vi "Example - Basic IPS-Use_In_Loops.vi"(0 "Connection Details":T5={"VISA resource name"="", "Comms Layer"=enum."Ethernet TCP/IP", "IP Address"="", "Serial Configuration"={"Baud Rate"=9600, "Parity"=0, "Data Bits"=8, "Stop Bits"=10, "Flow Control"=0}, "ISOBUS address"=-1} {"Serial Configuration"."Flow Control" items=["None", "XON/XOFF", "RTS/CTS", "XON/XOFF & RTS/CTS", "DTR/DSR", "XON/XOFF & DTR/DSR"]; "Serial Configuration"."Stop Bits" items=["1.0"=10, "2.0"=20]; "Serial Configuration"."Data Bits" items=["7"=7, "8"=8]; "Serial Configuration"."Parity" items=["None", "Odd", "Even"]; "Serial Configuration"."Baud Rate" items=["300"=300, "600"=600, "1200"=1200, "2400"=2400, "4800"=4800, "9600"=9600, "19200"=19200]}, 1 "Axis Group":string(combo)="GRPZ", 2 "ID Query (True)":bool=TRUE, 3 "Clear Previous Connections (False)":bool, 4 "HOLD":bool, 6 "Ramp Controls":T7 {"Target Rate (T/min)" format="%_5g"; "Target Field (T)" format="%_5g"; "Target Rate (A/min)" format="%_5g"; "Target Current (A)" format="%_5g"}, 7 "AMP/TESLA":bool, 8 "Magnet Controls":T8, 9 "SWITCH\nHEATER":bool, 11 "Sw Delay (s)":dbl=30.0 caption="Time Target (s)") -> (10 "System Time":string, 12 "Device Details":T1, 13 "SW HTR\nCONFIRM":bool, 14 "Output Current (A)":dbl format="%.4g", 15 "Magnet Current (A)":dbl format="%.4g", 16 "Output Voltage (V)":dbl format="%.4g", 17 "Current/Field (A/T)":dbl caption="Current Field Factor (A/T)" format="%#.4f", 18 "PSU Act Stat 2":T9 caption="Mode Status", 19 "error out":errorcluster)   [LabVIEW 2013, in "Mercury iXX.lvlib"]
uses:
  <instrlib>/Mercury iXX/Mercury iXX.lvlib
  <instrlib>/Mercury iXX/Public/Libraries/Magnet/Configuration/Read/Output Configuration (Read).vi
  <instrlib>/Mercury iXX/Public/Libraries/Magnet.lvlib
  <instrlib>/Mercury iXX/Public/Libraries/Magnet/Open/Open Magnet Device.vi
  <instrlib>/Mercury iXX/Public/Libraries/Magnet/Signals/Set/Switch Heater No Check (Set).vi
  <instrlib>/Mercury iXX/Public/Libraries/System/Open/Open System.vi
  <instrlib>/Mercury iXX/Public/Libraries/System.lvlib
  <instrlib>/Mercury iXX/Public/Libraries/System/Read/Catalogue (Read).vi
  <instrlib>/Mercury iXX/Public/Libraries/Magnet/Configuration/Read/Current to Field Factor (Read).vi
  <instrlib>/Mercury iXX/Public/Libraries/Magnet/Signals/Read/Switch Heater Status (Read).vi
  <instrlib>/Mercury iXX/Public/Libraries/Magnet/Signals/Read/Current (Read).vi
  <instrlib>/Mercury iXX/Public/Libraries/Magnet/Signals/Read/Voltage (Read).vi
  <instrlib>/Mercury iXX/Public/Libraries/Magnet/Signals/Read/Persistant Current (Read).vi
  <instrlib>/Mercury iXX/Public/Libraries/System/Read/Time (Read).vi
  <instrlib>/Mercury iXX/Public/Libraries/Magnet/Configuration/Read/PSU Action Status (Read).vi
  <instrlib>/Mercury iXX/Public/Libraries/Magnet/Configuration/Set/PSU Action Status (Set).vi
  <instrlib>/Mercury iXX/Public/Libraries/Magnet/Signals/Set/Target Current (Set).vi
  <instrlib>/Mercury iXX/Public/Libraries/Magnet/Signals/Set/Target Current Rate (Set).vi
  <instrlib>/Mercury iXX/Public/Libraries/Magnet/Signals/Set/Target Field (Set).vi
  <instrlib>/Mercury iXX/Public/Libraries/Magnet/Signals/Set/Target Field Rate (Set).vi
  <instrlib>/Mercury iXX/Public/Libraries/Magnet/Controls/PSU Actions.ctl
  <instrlib>/Mercury iXX/Public/Libraries/Magnet/Controls/Switch Heater.ctl
  <instrlib>/Mercury iXX/Public/Controls/Comms Transport Layer.ctl
  <instrlib>/Mercury iXX/Public/Controls/Serial Settings.ctl
  <instrlib>/Mercury iXX/Public/Controls/ISOBus Address.ctl
  <instrlib>/Mercury iXX/Public/Libraries/Magnet/Controls/Output Configuration.ctl
panel:
  out "Switch Time":string
  in  "Tab Control":enum32{"Connection", "Front_Panel", "Error"}(tab)
  out "Number of Mag Units\nin the group":dbl
  out "Out Config 2":T6="PARA" caption="Output Configuration"
  out "Voltage (V)":dbl(knob) scale=-10.0..10.0
  out "Current (A)":dbl(knob) scale=-60.0..60.0
  out "Elapsed\nTime (s)":dbl caption="Elapsed Time (s)"
  out "Magnet Centre Field (T)":dbl format="%.4g"
  out "Output (T) (Field equivalent)":dbl format="%.4g"
  # "SWITCH CONTROLS"
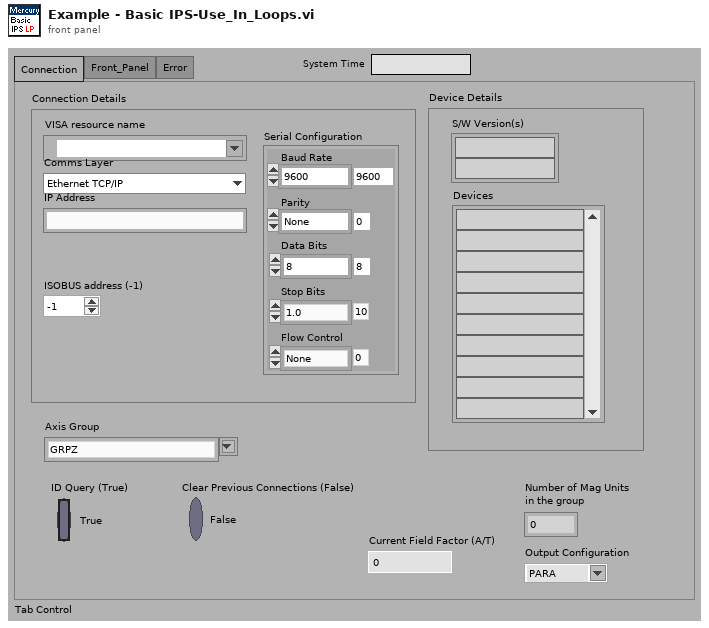
[diagram p1: front panel]
types:
  T1 = cluster{"Devices":string[], "S/W Version(s)":string[]}
  T2 = typedef "Mercury iXX.lvlib/Comms Transport Layer.ctl" = enum16{"Ethernet TCP/IP", "USB", "ISOBus - RS-232", "GPIB"}
  T3 = typedef "Mercury iXX.lvlib/Serial Settings.ctl" = cluster{"Baud Rate":u32, "Parity":u16, "Data Bits":u16, "Stop Bits":u16, "Flow Control":u16}
  T4 = typedef "Mercury iXX.lvlib/ISOBus Address.ctl" = i32
  T5 = cluster{"VISA resource name":refnum<visa-resource-name>, "Comms Layer":T2, "IP Address":string, "Serial Configuration":T3, "ISOBUS address":T4}
  T6 = typedef "Mercury iXX.lvlib/Magnet.lvlib/Output Configuration.ctl" = string
  T7 = cluster{"Target Current (A)":dbl, "Target Rate (A/min)":dbl, "SEND TO IPS":bool, "Target Field (T)":dbl, "Target Rate (T/min)":dbl}
  T8 = cluster{"CLAMP":bool, "TO SET":bool, "TO ZERO":bool}
  T9 = typedef "Mercury iXX.lvlib/Magnet.lvlib/PSU Actions.ctl" = string
  T10 = typedef "Mercury iXX.lvlib/Mercury Reference.ctl" = cluster{"Comms":refnum<visa-resource-name>, "Device ID":string[], "Comms Layer":T2, "Command":string, "Query reference":T11}
  T11 = typedef "Mercury iXX.lvlib/Query Dynamic Reference.ctl" = refnum<vi>
  T12 = typedef "Mercury iXX.lvlib/Magnet.lvlib/Switch Heater.ctl" = string
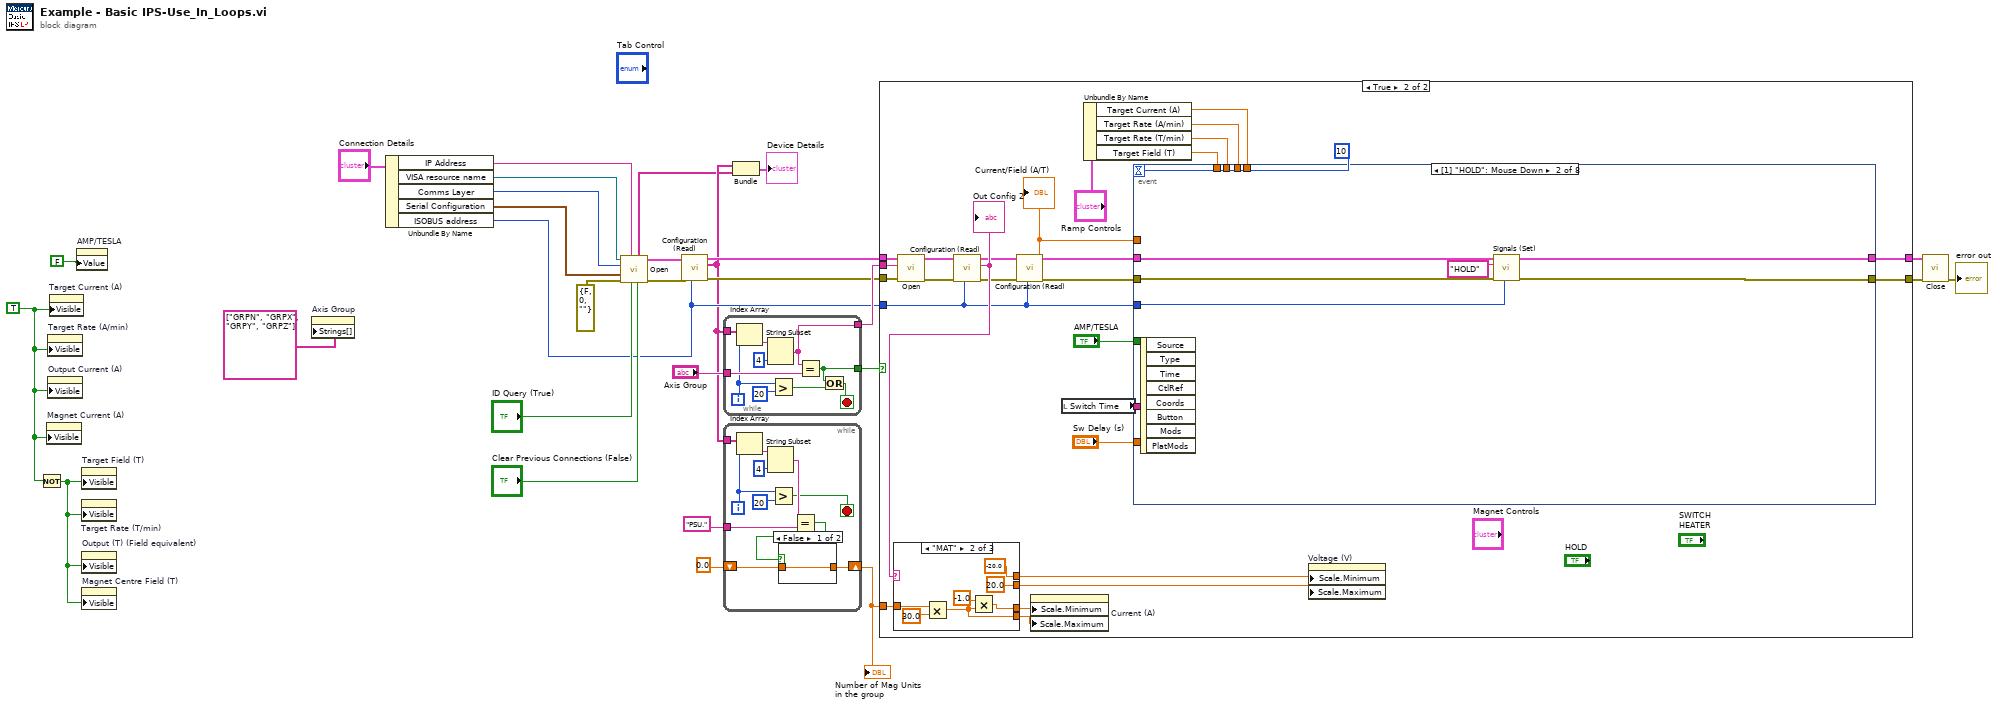
[diagram p0: block diagram]
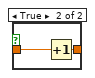
[diagram p2: hidden frame]
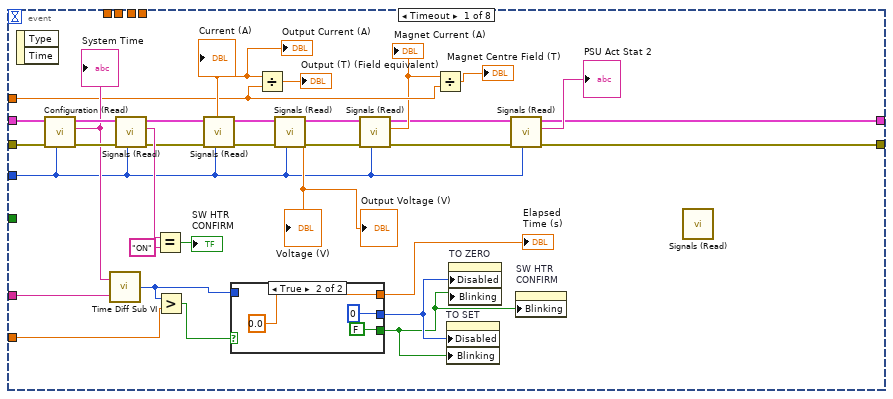
[diagram p4: hidden frame]
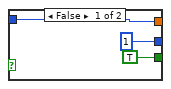
[diagram p5: hidden frame]
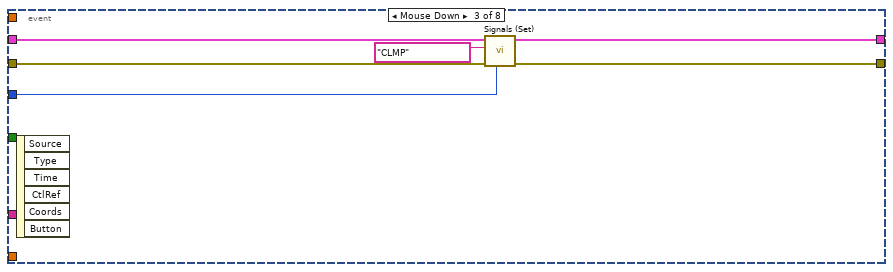
[diagram p6: hidden frame]
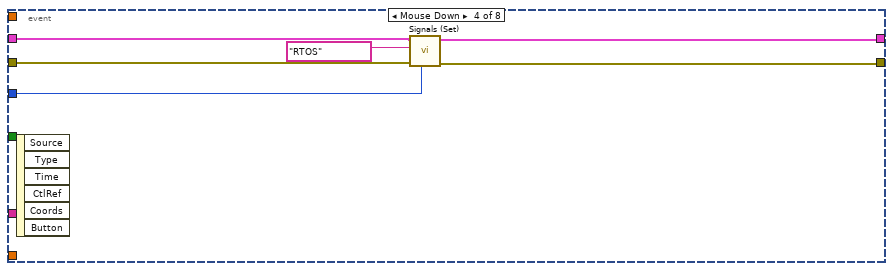
[diagram p7: hidden frame]
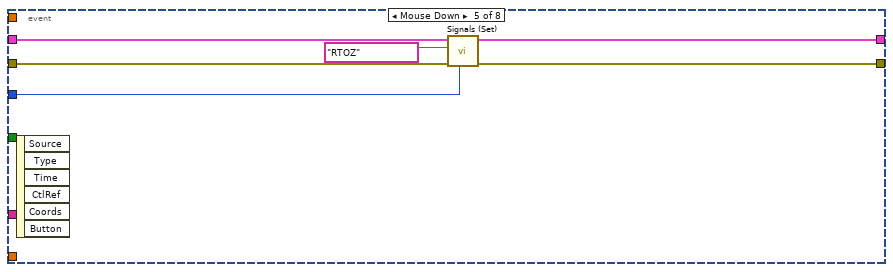
[diagram p8: hidden frame]
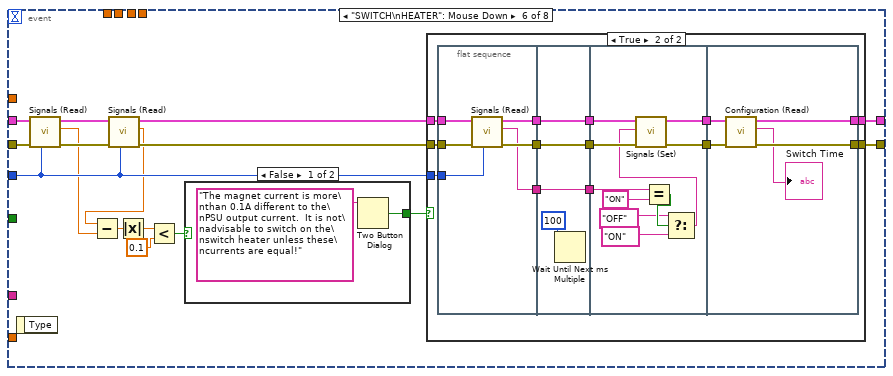
[diagram p9: hidden frame]
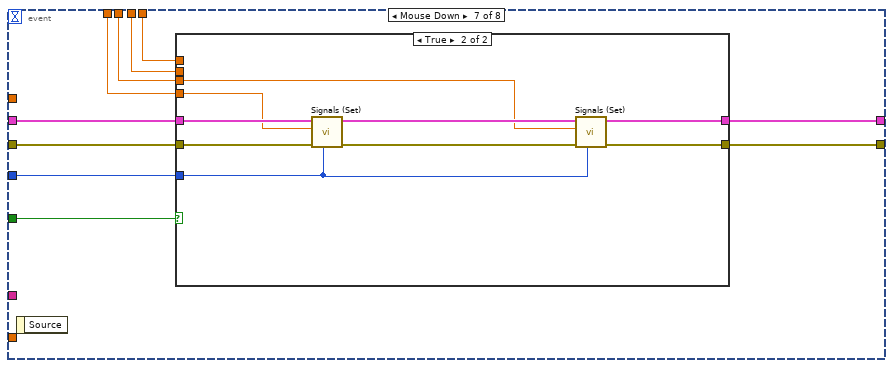
[diagram p12: hidden frame]
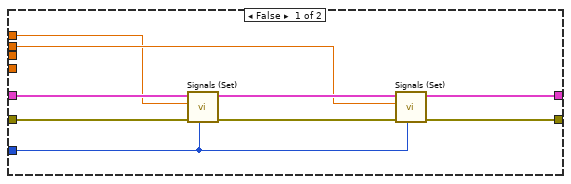
[diagram p13: hidden frame]
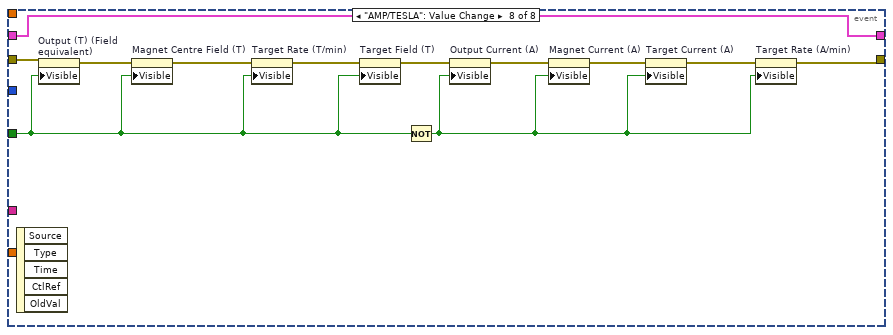
[diagram p14: hidden frame]
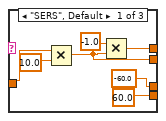
[diagram p15: hidden frame]
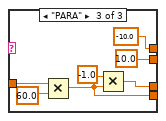
[diagram p16: hidden frame]
diagram:
  w11 = TRUE ("Visible")
  n1 = Not(x=w11) -> (.not. x?=w10:bool)
  n2 = property on="Magnet Current (A)" class="DigNum (strict)"("Visible"=w11) -> ()  [unwired: 2 in, 2 out]
  n3 = property on="Target Rate (A/min)" class="DigNum (strict)"("Visible"=w11) -> ()  [unwired: 2 in, 2 out]
  n4 = property on="Output Current (A)" class="DigNum (strict)"("Visible"=w11) -> ()  [unwired: 2 in, 2 out]
  n5 = property on="Target Current (A)" class="DigNum (strict)"("Visible"=w11) -> ()  [unwired: 2 in, 2 out]
  n6 = property on="AMP/TESLA" class="Bool (strict)"("Value"=FALSE ("AMP/TESLA")) -> ()  [unwired: 2 in, 2 out]
  n7 = property on="Target Field (T)" class="DigNum (strict)"("Visible"=w10) -> ()  [unwired: 2 in, 2 out]
  n8 = property on="Target Rate (T/min)" class="DigNum (strict)"("Visible"=w10) -> ()  [unwired: 2 in, 2 out]
  n9 = property on="Output (T) (Field equivalent)" class="DigNum (strict)"("Visible"=w10) -> ()  [unwired: 2 in, 2 out]
  n10 = property on="Magnet Centre Field (T)" class="DigNum (strict)"("Visible"=w10) -> ()  [unwired: 2 in, 2 out]
  n11 = property on="Axis Group" class="CmbBox"("Strings[]"=string[] ["GRPN", "GRPX", "GRPY", "GRPZ"]) -> ()  [unwired: 2 in, 2 out]
  n12 = Unbundle By Name("Connection Details") -> ("IP Address"=w6:string, "VISA resource name"=w5:refnum<visa-resource-name>, "Comms Layer"=w4:T2, "Serial Configuration"=w8:T3, "ISOBUS address"=w7:T4)
  n13 = call-poly <instrlib>:"Open.vi"("Clear Previous Connections (False)"="Clear Previous Connections (False)", "ID Query (True)"="ID Query (True)", "IP Address"=w6, "error in (no error)"=errorcluster {"status"=FALSE, "code"=0, "source"=""}, "Serial Configuration"=w8, "Comms Layer"=w4, "VISA resource name"=w5) -> ("error out"=w25:errorcluster, "Mercury Reference Out"=w26:T10, "S/W Version(s)"=w1:string[])  [unwired: 2 out]
  n14 = call-poly <instrlib>:"Configuration (Read).vi"("ISOBUS address"=w7, "error in"=w25, "Mercury Reference In"=w26) -> ("error out"=w13:errorcluster, "Devices"=w2:string[], "Mercury Reference Out"=w14:T10)  [unwired: 6 out]
  n15 = while {
    tunnel: w2 -> [w39]
    tunnel: [w30] -> w23
    tunnel: "Axis Group" -> [w36]
    tunnel: [w31] -> w24
    i -> [w34]
    stop <- w33 stop-if-true
    n16 = Index Array(array=w39, index=w34) -> (element=w37:string)
    n17 = String Subset(string=w37, length (rest)=4 ("length (rest)")) -> (substring=w30:string)  [unwired: 1 out]
    n18 = Greater?(x=w34, y=20) -> (0:w32:bool)
    n19 = Equal?(x=w30, y=w36) -> (x = y?=w31:bool)
    n20 = Or(x=w31, y=w32) -> (x .or. y?=w33:bool)
  }
  n21 = while {
    shift-right: [w46] -> w15
    shift-left: 0.0 -> [w45]
    tunnel: "PSU." -> [w42]
    tunnel: w2 -> [w41]
    i -> [w48]
    stop <- w43 stop-if-true
    n22 = Index Array(array=w41, index=w48) -> (element=w40:string)
    n23 = String Subset(string=w40, length (rest)=4 ("length (rest)")) -> (substring=w47:string)  [unwired: 1 out]
    n24 = Greater?(x=w48, y=20) -> (0:w43:bool)
    n25 = Equal?(x=w47, y=w42) -> (x = y?=w44:bool)
    n26 = case shown="False" w44 {
      tunnel: [w51 w53] -> w46
      tunnel: w45 -> [w51 w52]
      frame False {
      }
      frame True {
        n27 = Increment(x=w52) -> (x+1=w53:dbl)
      }
    }
  }
  "Number of Mag Units\nin the group" <- w15
  n28 = Bundle("Devices"=w2, "S/W Version(s)"=w1) -> (→"Device Details":T1)  [unwired: 1 out]
  n29 = case shown="True" w24 {
    tunnel: w14 -> [w55 w83]
    tunnel: w23 -> [_ w82]
    tunnel: w7 -> [_ w69]
    tunnel: [w55 w81] -> w22
    tunnel: [w54 w80] -> w21
    tunnel: w15 -> [_ w77]
    tunnel: w13 -> [w54 w66]
    frame False {
    }
    frame True {
      n30 = call-poly <instrlib>:"Open.vi"("error in (no error)"=w66, "Device Identifier"=w82, "Mercury Reference In"=w83) -> ("error out"=w78:errorcluster, "Mercury Reference Out"=w79:T10)  [unwired: 7 out]
      n31 = call-poly <instrlib>:"Configuration (Read).vi"("ISOBUS address"=w69, "error in"=w78, "Mercury Reference In"=w79) -> ("error out"=w71:errorcluster, "Out Config"=w76:T6, "Mercury Reference Out"=w70:T10)  [unwired: 6 out]
      "Out Config 2" <- w76
      n32 = case shown="\"MAT\"" w76 {
        tunnel: w77 -> [w248 w255 w264]
        tunnel: [60.0 ("y") w254 w261] -> w74
        tunnel: [-60.0 ("y") w253 w260] -> w75
        tunnel: [w247 -20.0 ("y") -10.0 ("y")] -> w73
        tunnel: [w246 20.0 ("y") 10.0 ("y")] -> w72
        frame "SERS", Default {
          n33 = Multiply(x=w248, y=10.0) -> (x*y=w246:dbl)
          n34 = Multiply(x=-1.0, y=w246) -> (x*y=w247:dbl)
        }
        frame "MAT" {
          n35 = Multiply(x=w255, y=30.0) -> (x*y=w254:dbl)
          n36 = Multiply(x=-1.0, y=w254) -> (x*y=w253:dbl)
        }
        frame "PARA" {
          n37 = Multiply(x=w264, y=60.0) -> (x*y=w261:dbl)
          n38 = Multiply(x=-1.0, y=w261) -> (x*y=w260:dbl)
        }
      }
      n39 = call-poly <instrlib>:"Configuration (Read).vi"("ISOBUS address"=w69, "error in"=w71, "Mercury Reference In"=w70) -> ("error out"=w68:errorcluster, "AtoB"=w65:dbl, "Mercury Reference Out"=w67:T10)  [unwired: 6 out]
      "Current/Field (A/T)" <- w65
      n40 = property on="Current (A)" class="Knob (strict)"("Scale.Minimum"=w75, "Scale.Maximum"=w74) -> ()  [unwired: 2 in, 2 out]
      n41 = local read "Switch Time"() -> (w63:string)
      n42 = Unbundle By Name("Ramp Controls") -> ("Target Current (A)"=w58:dbl, "Target Rate (A/min)"=w59:dbl, "Target Rate (T/min)"=w57:dbl, "Target Field (T)"=w56:dbl)
      n43 = event shown="[1] \"HOLD\": Mouse Down" {
        selector: _ -> [_ _ _ _ _ _ _ _]
        dyn-events: _ -> [_ _ _ _ _ _ _ _]
        timeout: 10 -> [_ _ _ _ _ _ _ _]
        tunnel: w67 -> [w114 w125 w132 w138 w144 w154 w213 w232]
        tunnel: w68 -> [w113 w126 w131 w137 w143 w153 w212 w243]
        tunnel: w69 -> [w87 w124 w128 w134 w142 w155 w211 _]
        tunnel: [w85 w123 w130 w136 w141 w160 w210 w232] -> w81
        tunnel: [w84 w122 w129 w135 w140 w159 w209 w235] -> w80
        tunnel: w63 -> [w101 _ _ _ _ _ _ _]
        tunnel: "Sw Delay (s)" -> [w100 _ _ _ _ _ _ _]
        tunnel: w65 -> [w91 _ _ _ _ _ _ _]
        tunnel: "AMP/TESLA" -> [_ _ _ _ _ _ w208 w234]
        tunnel: w59 -> [_ _ _ _ _ _ w207 _]
        tunnel: w58 -> [_ _ _ _ _ _ w206 _]
        tunnel: w57 -> [_ _ _ _ _ _ w205 _]
        tunnel: w56 -> [_ _ _ _ _ _ w204 _]
        event Timeout {
          n44 = event-data() -> ()  [unwired: 3 out]
          n45 = call-poly <instrlib>:"Signals (Read).vi"("ISOBUS address"=w87, "error in"=w113, "Mercury Reference In"=w114) -> ("error out"=w106:errorcluster, "Switch Heater Status"=w112:string, "Mercury Reference Out"=w109:T10)  [unwired: 6 out]
          n46 = Equal?(x=w112, y="ON") -> (x = y?=→"SW HTR\nCONFIRM":bool)
          n47 = call-poly <instrlib>:"Signals (Read).vi"("ISOBUS address"=w87, "error in"=w106, "Mercury Reference In"=w109) -> ("error out"=w105:errorcluster, "Current"=w93:dbl, "Mercury Reference Out"=w108:T10)  [unwired: 6 out]
          "Current (A)" <- w93
          "Output Current (A)" <- w93
          n48 = Divide(x=w93, y=w91) -> (x/y=→"Output (T) (Field equivalent)":dbl)
          n49 = call-poly <instrlib>:"Signals (Read).vi"("ISOBUS address"=w87, "error in"=w105, "Mercury Reference In"=w108) -> ("error out"=w104:errorcluster, "Voltage"=→"Voltage (V)" →"Output Voltage (V)":dbl, "Mercury Reference Out"=w107:T10)  [unwired: 6 out]
          n50 = call-poly <instrlib>:"Signals (Read).vi"("ISOBUS address"=w87, "error in"=w104, "Mercury Reference In"=w107) -> ("error out"=w88:errorcluster, "Persistant Current"=w90:dbl, "Mercury Reference Out"=w89:T10)  [unwired: 6 out]
          "Magnet Current (A)" <- w90
          n51 = call-poly <instrlib>:"Configuration (Read).vi"("ISOBUS address"=w87, "error in"=w88, "Mercury Reference In"=w89) -> ("Time"=w102:string)  [unwired: 8 out]
          "System Time" <- w102
          n52 = call <instrlib>:"Time Diff Sub VI.vi"("Start Time (hh:mm:ss)"=w101, "Current Time (hh:mm:ss)"=w102) -> ("Time Diff (s)"=w97:i32)
          n53 = Greater?(x=w97, y=w100) -> (0:w99:bool)
          n54 = case shown="True" w99 {
            tunnel: [w117 0.0 ("Elapsed\nTime (s)")] -> w98
            tunnel: w97 -> [w117 _]
            tunnel: [TRUE ("Blinking") FALSE ("Blinking")] -> w95
            tunnel: [u8 1 ("Disabled") u8 0 ("Disabled")] -> w96
            frame False {
            }
            frame True {
            }
          }
          "Elapsed\nTime (s)" <- w98
          n55 = Divide(x=w90, y=w91) -> (x/y=→"Magnet Centre Field (T)":dbl)
          n56 = property on="TO SET" class="Bool"("Disabled"=w96, "Blinking"=w95) -> ()  [unwired: 2 in, 2 out]
          n57 = property on="TO ZERO" class="Bool"("Disabled"=w96, "Blinking"=w95) -> ()  [unwired: 2 in, 2 out]
          n58 = call-poly <instrlib>:"Signals (Read).vi"("ISOBUS address"=w87, "error in"=w88, "Mercury Reference In"=w89) -> ("error out"=w84:errorcluster, "PSU Act Stat"=→"PSU Act Stat 2":T9, "Mercury Reference Out"=w85:T10)  [unwired: 6 out]
          n59 = property on="SW HTR\nCONFIRM" class="Bool (strict)"("Blinking"=w95) -> ()  [unwired: 2 in, 2 out]
          n60 = call-poly <instrlib>:"Signals (Read).vi"() -> ()  [unwired: 3 in, 9 out]
        }
        event "HOLD": Mouse Down {
          n61 = event-data() -> ()  [unwired: 9 out]
          n62 = call-poly <instrlib>:"Signals (Set).vi"("ISOBUS address"=w124, "error in"=w126, "PSU Act Stat"=T9 "HOLD", "Mercury Reference In"=w125) -> ("error out"=w122:errorcluster, "Mercury Reference Out"=w123:T10)  [unwired: 6 out]
        }
        event "Magnet Controls.CLAMP": Mouse Down {
          n63 = event-data() -> ()  [unwired: 7 out]
          n64 = call-poly <instrlib>:"Signals (Set).vi"("ISOBUS address"=w128, "error in"=w131, "PSU Act Stat"=T9 "CLMP", "Mercury Reference In"=w132) -> ("error out"=w129:errorcluster, "Mercury Reference Out"=w130:T10)  [unwired: 6 out]
        }
        event "Magnet Controls.TO SET": Mouse Down {
          n65 = event-data() -> ()  [unwired: 7 out]
          n66 = call-poly <instrlib>:"Signals (Set).vi"("ISOBUS address"=w134, "error in"=w137, "PSU Act Stat"=T9 "RTOS", "Mercury Reference In"=w138) -> ("error out"=w135:errorcluster, "Mercury Reference Out"=w136:T10)  [unwired: 6 out]
        }
        event "Magnet Controls.TO ZERO": Mouse Down {
          n67 = event-data() -> ()  [unwired: 7 out]
          n68 = call-poly <instrlib>:"Signals (Set).vi"("ISOBUS address"=w142, "error in"=w143, "PSU Act Stat"=T9 "RTOZ", "Mercury Reference In"=w144) -> ("error out"=w140:errorcluster, "Mercury Reference Out"=w141:T10)  [unwired: 6 out]
        }
        event "SWITCH\nHEATER": Mouse Down {
          n69 = event-data() -> ()  [unwired: 2 out]
          n70 = call-poly <instrlib>:"Signals (Read).vi"("ISOBUS address"=w155, "error in"=w153, "Mercury Reference In"=w154) -> ("error out"=w156:errorcluster, "Current"=w149:dbl, "Mercury Reference Out"=w157:T10)  [unwired: 6 out]
          n71 = call-poly <instrlib>:"Signals (Read).vi"("ISOBUS address"=w155, "error in"=w156, "Mercury Reference In"=w157) -> ("error out"=w152:errorcluster, "Persistant Current"=w150:dbl, "Mercury Reference Out"=w151:T10)  [unwired: 6 out]
          n72 = Subtract(x=w150, y=w149) -> (x-y=w148:dbl)
          n73 = Absolute Value(x=w148) -> (abs(x)=w147:dbl)
          n74 = Less?(x=w147, y=0.1) -> (x < y?=w145:bool)
          n75 = case shown="False" w145 {
            selector: w145 -> [_ w163]
            tunnel: [w162 w163] -> w158
            frame False {
              n76 = Two Button Dialog(message="The magnet current is more\nthan 0.1A different to the\nPSU output current.  It is not\nadvisable to switch on the\nswitch heater unless these\ncurrents are equal!") -> (T button?=w162:bool)  [unwired: 2 out]
            }
            frame True {
            }
          }
          n77 = case shown="True" w158 {
            tunnel: w151 -> [w165 w170]
            tunnel: w152 -> [w164 w169]
            tunnel: w155 -> [_ w168]
            tunnel: [w165 w167] -> w160
            tunnel: [w164 w166] -> w159
            frame False {
            }
            frame True {
              n78 = flat-sequence {
                tunnel: [w181] -> w178
                tunnel: [w180] -> w177
                tunnel: [w179] -> w176
                tunnel: w170 -> [w184]
                tunnel: w169 -> [w183]
                tunnel: w168 -> [w182]
                tunnel: w178 -> [w187]
                tunnel: w177 -> [w186]
                tunnel: [w187] -> w175
                tunnel: [w186] -> w174
                tunnel: [w185] -> w173
                tunnel: w176 -> [w185]
                tunnel: w175 -> [w197]
                tunnel: w174 -> [w198]
                tunnel: w173 -> [w195]
                tunnel: [w192] -> w172
                tunnel: [w193] -> w171
                tunnel: w172 -> [w203]
                tunnel: w171 -> [w202]
                tunnel: [w201] -> w167
                tunnel: [w200] -> w166
                frame #0 {
                  n79 = call-poly <instrlib>:"Signals (Read).vi"("ISOBUS address"=w182, "error in"=w183, "Mercury Reference In"=w184) -> ("error out"=w181:errorcluster, "Switch Heater Status"=w179:string, "Mercury Reference Out"=w180:T10)  [unwired: 6 out]
                }
                frame #1 {
                  n80 = Wait Until Next ms Multiple(millisecond multiple=u32 100) -> ()  [unwired: 1 out]
                }
                frame #2 {
                  n81 = Equal?(x=w195, y="ON") -> (x = y?=w194:bool)
                  n82 = Select(t=T12 "OFF" ("Set Switch Heater"), s=w194, f=T12 "ON" ("Set Switch Heater")) -> (s? t:f=w189:T12)
                  n83 = call-poly <instrlib>:"Signals (Set).vi"("error in"=w197, "Set Switch Heater"=w189, "Mercury Reference In"=w198) -> ("error out"=w193:errorcluster, "Mercury Reference Out"=w192:T10)  [unwired: 1 in, 6 out]
                }
                frame #3 {
                  n84 = call-poly <instrlib>:"Configuration (Read).vi"("error in"=w202, "Mercury Reference In"=w203) -> ("error out"=w200:errorcluster, "Time"=→"Switch Time":string, "Mercury Reference Out"=w201:T10)  [unwired: 1 in, 6 out]
                }
              }
            }
          }
        }
        event "Ramp Controls.SEND TO IPS": Mouse Down {
          n85 = event-data() -> ()  [unwired: 2 out]
          n86 = case shown="True" w208 {
            tunnel: w213 -> [w222 w231]
            tunnel: w212 -> [w221 w230]
            tunnel: w211 -> [w218 w225]
            tunnel: [w217 w227] -> w210
            tunnel: [w216 w226] -> w209
            tunnel: w207 -> [w215 _]
            tunnel: w206 -> [w214 _]
            tunnel: w205 -> [_ w224]
            tunnel: w204 -> [_ w223]
            frame False {
              n87 = call-poly <instrlib>:"Signals (Set).vi"("ISOBUS address"=w218, "error in"=w221, "Target Current"=w214, "Mercury Reference In"=w222) -> ("error out"=w219:errorcluster, "Mercury Reference Out"=w220:T10)  [unwired: 1 in, 5 out]
              n88 = call-poly <instrlib>:"Signals (Set).vi"("ISOBUS address"=w218, "error in"=w219, "Target Current Rate"=w215, "Mercury Reference In"=w220) -> ("error out"=w216:errorcluster, "Mercury Reference Out"=w217:T10)  [unwired: 1 in, 5 out]
            }
            frame True {
              n89 = call-poly <instrlib>:"Signals (Set).vi"("ISOBUS address"=w225, "error in"=w230, "Target Field"=w223, "Mercury Reference In"=w231) -> ("error out"=w228:errorcluster, "Mercury Reference Out"=w229:T10)  [unwired: 1 in, 5 out]
              n90 = call-poly <instrlib>:"Signals (Set).vi"("ISOBUS address"=w225, "error in"=w228, "Target Field Rate"=w224, "Mercury Reference In"=w229) -> ("error out"=w226:errorcluster, "Mercury Reference Out"=w227:T10)  [unwired: 1 in, 5 out]
            }
          }
        }
        event "AMP/TESLA": Value Change {
          n91 = event-data() -> ()  [unwired: 6 out]
          n92 = property on="Output (T) (Field equivalent)" class="DigNum (strict)"(error in=w243, "Visible"=w234) -> (error out=w242:errorcluster)  [unwired: 1 in, 1 out]
          n93 = property on="Magnet Centre Field (T)" class="DigNum (strict)"(error in=w242, "Visible"=w234) -> (error out=w241:errorcluster)  [unwired: 1 in, 1 out]
          n94 = property on="Target Rate (T/min)" class="DigNum (strict)"(error in=w241, "Visible"=w234) -> (error out=w240:errorcluster)  [unwired: 1 in, 1 out]
          n95 = property on="Target Field (T)" class="DigNum (strict)"(error in=w240, "Visible"=w234) -> (error out=w239:errorcluster)  [unwired: 1 in, 1 out]
          n96 = Not(x=w234) -> (.not. x?=w233:bool)
          n97 = property on="Output Current (A)" class="DigNum (strict)"(error in=w239, "Visible"=w233) -> (error out=w238:errorcluster)  [unwired: 1 in, 1 out]
          n98 = property on="Magnet Current (A)" class="DigNum (strict)"(error in=w238, "Visible"=w233) -> (error out=w237:errorcluster)  [unwired: 1 in, 1 out]
          n99 = property on="Target Current (A)" class="DigNum (strict)"(error in=w237, "Visible"=w233) -> (error out=w236:errorcluster)  [unwired: 1 in, 1 out]
          n100 = property on="Target Rate (A/min)" class="DigNum (strict)"(error in=w236, "Visible"=w233) -> (error out=w235:errorcluster)  [unwired: 1 in, 1 out]
        }
      }
      n101 = property on="Voltage (V)" class="Knob (strict)"("Scale.Minimum"=w73, "Scale.Maximum"=w72) -> ()  [unwired: 2 in, 2 out]
    }
  }
  n102 = call <instrlib>:"Close.vi"("error in (no error)"=w21, "Mercury Reference"=w22) -> ("error out"=→"error out":errorcluster)  [unwired: 9 out]
